vi "test Deployment Cluster Configuration.vi"(8 "error in":errorcluster, 11 "TestCase in":refnum<class "Deployment.lvclass">) -> (0 "error out":errorcluster, 3 "TestCase out":refnum<class "Deployment.lvclass">)   [LabVIEW 2020, in "Deployment.lvclass"]
uses:
  Deployment.lvclass
  Shared/1553 Channel.ctl
  Shared/Terminal Name and Address.ctl
  Shared/Address.ctl
  Shared/Message Definition.ctl
  Shared/Message Type.ctl
  Shared/Terminal Endpoint.ctl
  Shared/Parameter Definition.ctl
  Deployment.lvclass/Deployment.ctl
  315b1c3a-44c8-49e8-b756-01f865c29b4a.vi
  <vilib>/addons/_JKI Toolkits/VI Tester/TestCase.llb/TestCase.lvclass
  niveristand-custom-device-testing-tools/VeriStandTestUtilities/VeriStandTestUtilities.lvlib
  Scripting/Ballard MIL-STD-1553 Scripting.lvlib
  C:/Program Files (x86)/National Instruments/LabVIEW 2020/vi.lib/addons/_JKI Toolkits/VI Tester/TestCase.llb/TestCase.lvclass
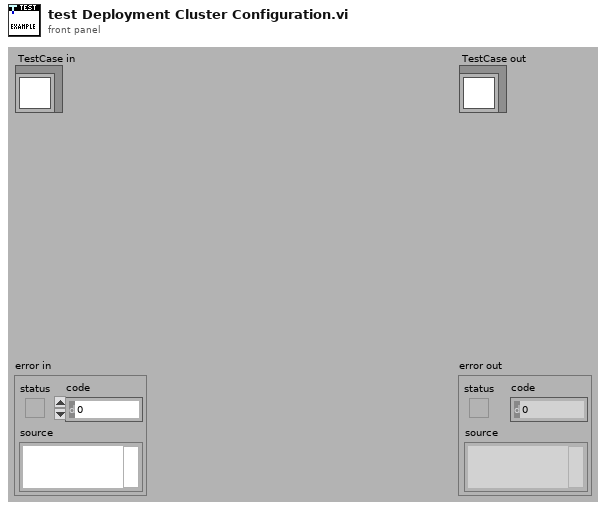
[diagram p1: front panel]
types:
  T1 = typedef "1553 Channel.ctl" = cluster{"HW channel":u16, "terminals":T2[], "messages":T4[], "acyclic frame names":string[]}
  T2 = typedef "Terminal Name and Address.ctl" = cluster{"name":string, "terminal address":T3}
  T3 = typedef "Address.ctl" = u16
  T4 = typedef "Message Definition.ctl" = cluster{"name":string, "message type":T5, "endpoint Rx":T6, "endpoint Tx":T6, "mode code":u16, "number of words":u16, "parameters":cluster{"name":string, "default value":dbl, "unit":string, "parameter definition":T7}[], "create timestamp channel":bool}
  T5 = typedef "Message Type.ctl" = string
  T6 = typedef "Terminal Endpoint.ctl" = cluster{"terminal address":T3, "subaddress":T3}
  T7 = typedef "Parameter Definition.ctl" = cluster{"start index":i32, "size (bits)":i32, "encoding":enum16{"BNR", "BCD", "Discrete"}, "signed":bool, "multiplier":dbl, "offset":dbl}
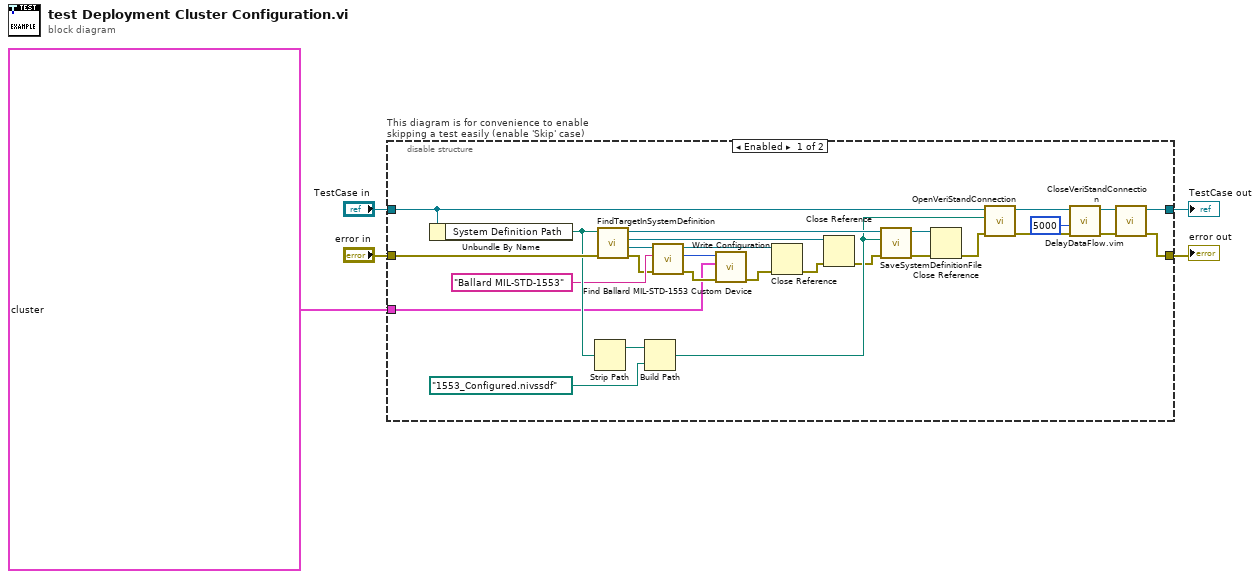
[diagram p0: block diagram]
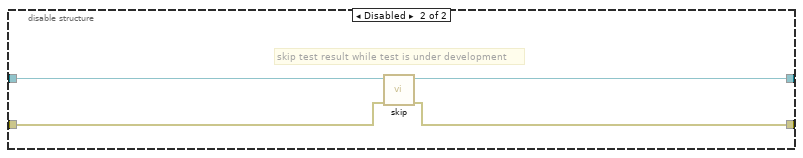
[diagram p2: hidden frame]
diagram:
  n1 = disable-structure "This diagram is for convenience to enable skipping a test easily (enable 'Skip' case)" shown="Enabled" {
    disable-tunnel: "TestCase in" -> [w26 w36]
    disable-tunnel: [w27 w34] -> w2
    disable-tunnel: [w29 w35] -> w4
    disable-tunnel: "error in" -> [w25 w33]
    disable-tunnel: T1[] [{"HW channel"=0, "terminals"=[{"name"="Bus Controller", "terminal address"=0}, {"name"="Remote Terminal 1", "terminal address"=1}, {"name"="Remote Terminal 15", "terminal address"=15}, {"name"="Remote Terminal 21", "terminal address"=21}, {"name"="Remote Terminal 31 (Broadcast)", "terminal address"=31}], "messages"=[{"name"="BC to RT 1.2", "message type"="BC to RT", "endpoint Rx"={"terminal address"=1, "subaddress"=2}, "endpoint Tx"={"terminal address"=0, "subaddress"=0}, "mode code"=0, "number of words"=3, "parameters"=[], "create timestamp channel"=FALSE}, {"name"="RT 31.15 to RT 21.21", "message type"="RT to RT", "endpoint Rx"={"terminal address"=31, "subaddress"=21}, "endpoint Tx"={"terminal address"=15, "subaddress"=21}, "mode code"=0, "number of words"=11, "parameters"=[], "create timestamp channel"=FALSE}, {"name"="BC to RT 3.0", "message type"="BC to RT", "endpoint Rx"={"terminal address"=1, "subaddress"=3}, "endpoint Tx"={"terminal address"=0, "subaddress"=0}, "mode code"=0, "number of words"=4, "parameters"=[], "create timestamp channel"=FALSE}, {"name"="RT 1.5 to BC", "message type"="RT to BC", "endpoint Rx"={"terminal address"=0, "subaddress"=0}, "endpoint Tx"={"terminal address"=1, "subaddress"=5}, "mode code"=0, "number of words"=6, "parameters"=[], "create timestamp channel"=FALSE}, {"name"="RT 1.6 to BC", "message type"="RT to BC", "endpoint Rx"={"terminal address"=0, "subaddress"=0}, "endpoint Tx"={"terminal address"=1, "subaddress"=6}, "mode code"=0, "number of words"=2, "parameters"=[], "create timestamp channel"=FALSE}, {"name"="RT 15.20 to RT 1.20", "message type"="RT to RT", "endpoint Rx"={"terminal address"=15, "subaddress"=20}, "endpoint Tx"={"terminal address"=1, "subaddress"=20}, "mode code"=0, "number of words"=4, "parameters"=[], "create timestamp channel"=FALSE}, {"name"="MC 16", "message type"="MC", "endpoint Rx"={"terminal address"=0, "subaddress"=0}, "endpoint Tx"={"terminal address"=1, "subaddress"=31}, "mode code"=16, "number of words"=1, "parameters"=[], "create timestamp channel"=FALSE}, {"name"="MC 17", "message type"="MC", "endpoint Rx"={"terminal address"=1, "subaddress"=31}, "endpoint Tx"={"terminal address"=0, "subaddress"=0}, "mode code"=17, "number of words"=1, "parameters"=[], "create timestamp channel"=FALSE}, {"name"="BC to RT 31.28", "message type"="BC to RT", "endpoint Rx"={"terminal address"=31, "subaddress"=28}, "endpoint Tx"={"terminal address"=0, "subaddress"=0}, "mode code"=0, "number of words"=6, "parameters"=[], "create timestamp channel"=FALSE}, {"name"="MC 1", "message type"="MC", "endpoint Rx"={"terminal address"=31, "subaddress"=31}, "endpoint Tx"={"terminal address"=0, "subaddress"=0}, "mode code"=1, "number of words"=0, "parameters"=[], "create timestamp channel"=FALSE}], "acyclic frame names"=["acyclicFrame ID56"]}] -> [w7 _]
    frame Enabled {
      n2 = Unbundle By Name(w26) -> ("System Definition Path"=w23:path)
      n3 = Strip Path(path=w23) -> (stripped path=w22:path)  [unwired: 1 out]
      n4 = call "FindTargetInSystemDefinition.vi"("error in"=w25, "system definition path"=w23) -> ("error out"=w10:errorcluster, "Target"=w13:refnum<k24>, "Root"=w16:refnum<k24>, "System Definition"=w24:refnum<k24>)  [unwired: 6 in]
      n5 = Build Path(base path=w22, name or relative path=path "1553_Configured.nivssdf") -> (appended path=w17:path)
      n6 = call "Find Ballard MIL-STD-1553 Custom Device.vi"("error in"=w10, "name"="Ballard MIL-STD-1553", "target in"=w13) -> ("error out"=w8:errorcluster, "custom device"=w9:u64, "target out"=w11:refnum<k24>)  [unwired: 6 in]
      n7 = call "Write Configuration.vi"("error in"=w8, "1553 channels"=w7, "Ballard MIL-STD 1553 custom device in"=w9) -> ("error out"=w6:errorcluster)  [unwired: 7 in, 1 out]
      n8 = Close Reference(reference=w11, error in (no error)=w6) -> (error out=w14:errorcluster)
      n9 = Close Reference(reference=w16, error in (no error)=w14) -> (error out=w15:errorcluster)
      n10 = call "SaveSystemDefinitionFile.vi"("error in (no error)"=w15, "System Definition File in"=w17, "System Definition Reference in"=w24) -> ("error out"=w19:errorcluster, "System Definition Reference out"=w20:refnum<k24>)  [unwired: 7 in]
      n11 = Close Reference(reference=w20, error in (no error)=w19) -> (error out=w18:errorcluster)
      n12 = call-dynamic "OpenVeriStandConnection.vi"("error in (no error)"=w18, "System Definition File"=w17, "VeriStand Test Case in"=w26) -> ("error out"=w32:errorcluster, "VeriStand Test Case out"=w28:refnum<class "Deployment.lvclass">)  [unwired: 6 in, 1 out]
      n13 = call "DelayDataFlow.vim"("value in"=w32, "milliseconds to wait"=u32 5000) -> ("value out"=w30:errorcluster)  [unwired: 2 in, 1 out]
      n14 = call-dynamic "CloseVeriStandConnection.vi"("error in (no error)"=w30, "VeriStand Test Case in"=w28) -> ("error out"=w29:errorcluster, "VeriStand Test Case out"=w27:refnum<class "Deployment.lvclass">)  [unwired: 8 in]
    }
    frame Disabled {
      # "skip test result while test is under development"
      n15 = call <vilib>:"skip.vi"("error in (no error)"=w33, "TestCase in"=w36) -> ("error out"=w35:errorcluster, "TestCase out"=w34:refnum<class "Deployment.lvclass">)  [unwired: 8 in]
    }
  }
  "error out" <- w4
  "TestCase out" <- w2
